vi "RT get system status.vi"(8 "error in (no error)":errorcluster, 9 "FPGA version":string="N/A", 10 "RT Main version":string="N/A", 11 "FPGA VI Reference in":refnum<k20>) -> (0 "error out":errorcluster, 3 "status summary string":string)   [LabVIEW 2018]
uses:
  Message Queue/error queue name (constant).ctl
  <vilib>/Utility/error.llb/Error Cluster From Error Code.vi
  <vilib>/rvi/errors/niLvFpgaAdjustHostInterfaceError.vi
  <vilib>/nisyscfg/Close (System).vi
  Globals/RT AND FPGA SETTINGS.vi
  <vilib>/rvi/interface/nirviReadWriteControl/nirviReadWriteControl.xnode
  <vilib>/NI_Real-Time Target Support.lvlib
  <vilib>/nisyscfg/nisyscfg.lvlib
  Message Queue/Message Queue.lvlib
  <resource>/objmgr/nisysapi.rc
  NiFpgaLv.dll
  <vilib>/rvi/interface/Simulation/niFpgaSimulationCallBeginRW.vi
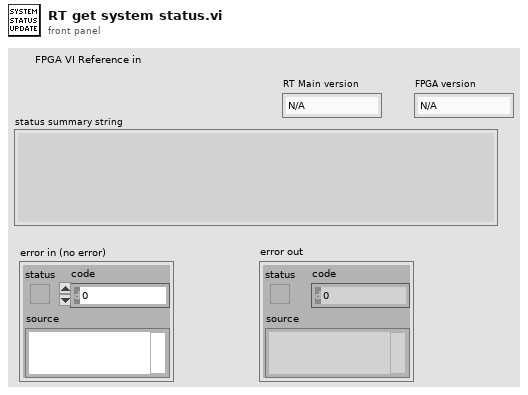
[diagram p1: front panel]
types:
  T1 = typedef "Message Queue.lvlib/error queue name (constant).ctl" = string
  T2 = enum16{"Safe State", "I/O with PID Control", "Fast Output Only", "NOT_READY"}
  T3 = typedef "NI_Real-Time Target Support.lvlib/RT CPU Load.ctl" = cluster{"Total (%)":dbl, "Time Critical (%)":dbl, "Timed Structures (%)":dbl, "High (%)":dbl, "Above Normal (%)":dbl, "Normal (%)":dbl, "Background (%)":dbl, "Idle (%)":dbl, "ISR (%)":dbl}
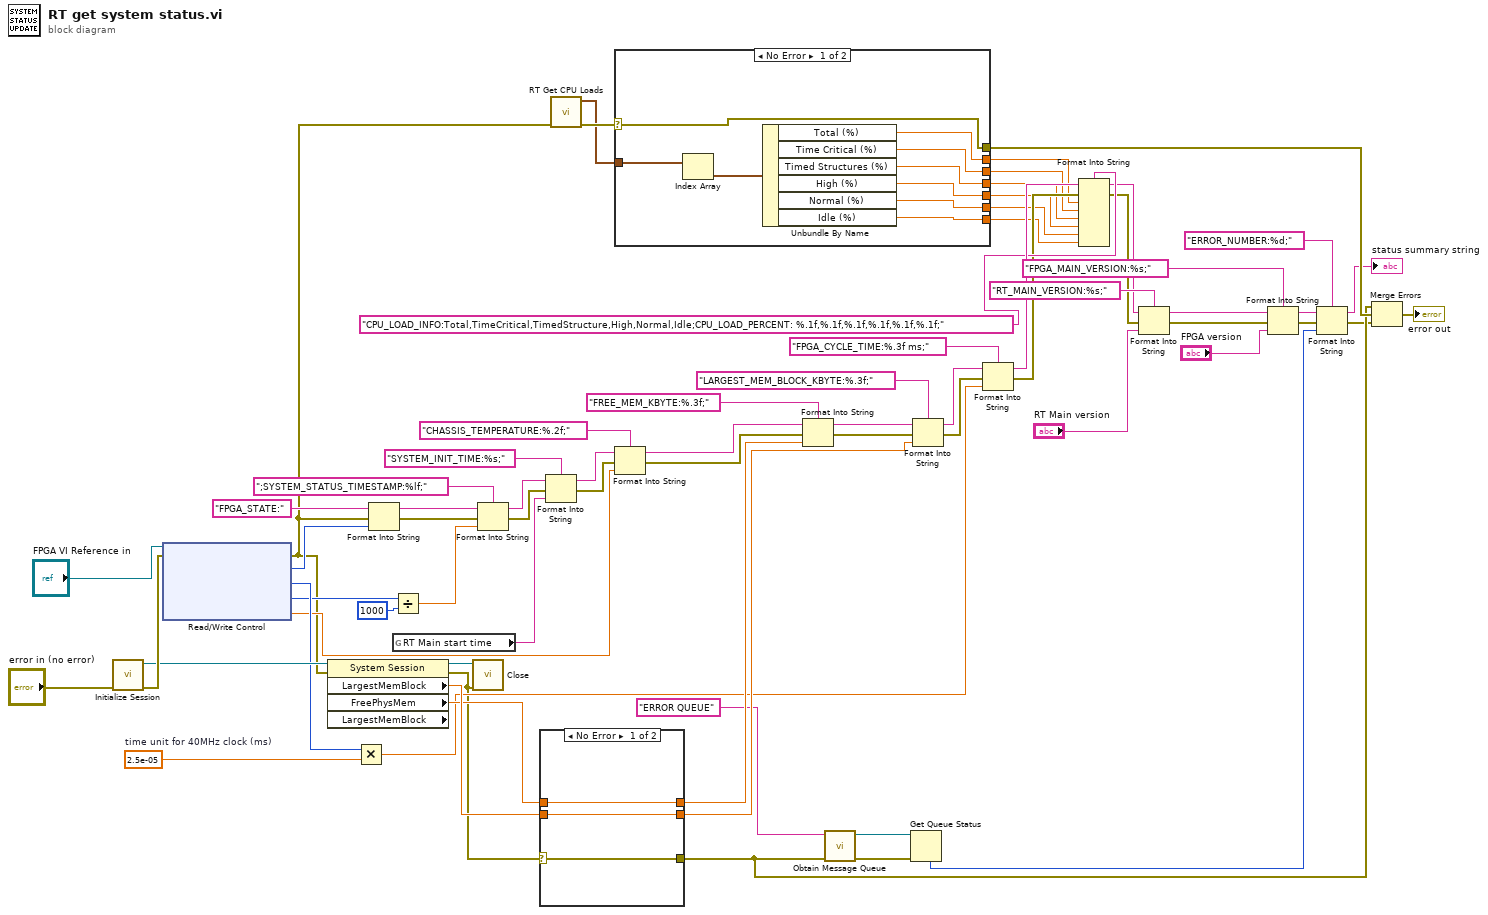
[diagram p0: block diagram]
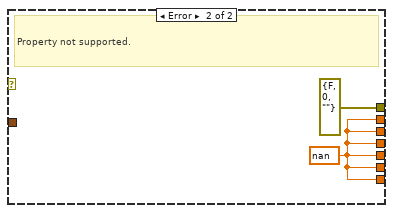
[diagram p2: hidden frame]
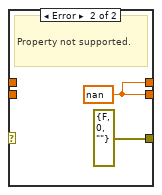
[diagram p3: hidden frame]
diagram:
  w56 = 2.5e-05  # time unit for 40MHz clock (ms)
  n1 = call <vilib>:"Initialize Session.vi"("error in (no error)"="error in (no error)") -> ("error out"=w70:errorcluster, "Session out"=w69:refnum<k21>)  [unwired: 9 in]
  n2 = xnode "Read/Write Control"("FPGA VI Reference In"="FPGA VI Reference in", "error in"=w70) -> ("error out"=w27:errorcluster, "FPGA state"=w65:T2, "ticks"=w57:i64, "time stamp (ms)"=w49:u64, "Chassis Temperature"=w44:sgl)  [unwired: 1 out]
  n3 = property class="System Session" props=["LargestMemBlock", "FreePhysMem", "LargestMemBlock"](reference=w69, error in=w27) -> (reference out=w8:refnum<k21>, error out=w7:errorcluster, "LargestMemBlock"=w67:dbl, "FreePhysMem"=w66:dbl)  [unwired: 1 out]
  n4 = Multiply(x=w57, y=w56) -> (x*y=w55:dbl)
  n5 = Format Into String(initial string="FPGA_STATE:", error in=w27, w65) -> (resulting string=w45:string, error out=w26:errorcluster)  [unwired: 1 in]
  n6 = Divide(x=w49, y=u64 1000) -> (x/y=w47:dbl)
  n7 = global read "RT AND FPGA SETTINGS.vi" "RT Main start time"() -> (w5:string)
  n8 = call-poly <vilib>:"Close.vi"("error in (no error)"=w7, "Session in"=w8) -> ()  [unwired: 9 in, 1 out]
  n9 = Format Into String(format string=";SYSTEM_STATUS_TIMESTAMP:%lf;", initial string=w45, error in=w26, w47) -> (resulting string=w2:string, error out=w4:errorcluster)
  n10 = case shown="No Error" w7 {
    selector: w7 -> [w71 _]
    tunnel: w67 -> [w72 _]
    tunnel: [w72 w75] -> w59
    tunnel: w66 -> [w73 _]
    tunnel: [w73 w75] -> w63
    tunnel: [w71 errorcluster {"status"=FALSE, "code"=0, "source"=""} ("error IO")] -> w33
    frame No Error {
    }
    frame Error {
      w75 = nan
      # "Property not supported."
    }
  }
  n11 = Format Into String(format string="SYSTEM_INIT_TIME:%s;", initial string=w2, error in=w4, w5) -> (resulting string=w1:string, error out=w3:errorcluster)
  n12 = call <vilib>:"RT Get CPU Loads.vi"("error in (no error)"=w27) -> ("error out"=w51:errorcluster, "CPU loads"=w50:T3[])  [unwired: 9 in]
  n13 = case shown="No Error" w51 {
    selector: w51 -> [w84 _]
    tunnel: [w81 w85] -> w15
    tunnel: [w84 errorcluster {"status"=FALSE, "code"=0, "source"=""} ("error IO")] -> w35
    tunnel: w50 -> [w82 _]
    tunnel: [w80 w85] -> w13
    tunnel: [w79 w85] -> w12
    tunnel: [w78 w85] -> w11
    tunnel: [w77 w85] -> w10
    tunnel: [w76 w85] -> w14
    frame No Error {
      n14 = Index Array(array=w82) -> (element=w83:T3)  [unwired: 1 in]
      n15 = Unbundle By Name(w83) -> ("Total (%)"=w81:dbl, "Time Critical (%)"=w76:dbl, "Timed Structures (%)"=w80:dbl, "High (%)"=w79:dbl, "Normal (%)"=w78:dbl, "Idle (%)"=w77:dbl)
    }
    frame Error {
      w85 = nan
      # "Property not supported."
    }
  }
  n16 = Format Into String(format string="CHASSIS_TEMPERATURE:%.2f;", initial string=w1, error in=w3, w44) -> (resulting string=w42:string, error out=w25:errorcluster)
  n17 = Format Into String(format string="FREE_MEM_KBYTE:%.3f;", initial string=w42, error in=w25, w63) -> (resulting string=w61:string, error out=w24:errorcluster)
  n18 = call "Obtain Message Queue.vi"("error in (no error)"=w33, "name (unnamed)"=T1 "ERROR QUEUE" ("Error queue name")) -> ("error out"=w32:errorcluster, "Message Queue"=w31:refnum<queue>)  [unwired: 7 in, 1 out]
  n19 = Get Queue Status(queue=w31, error in (no error)=w32) -> (# elements in queue=w30:i32)  [unwired: 1 in, 7 out]
  n20 = Format Into String(format string="LARGEST_MEM_BLOCK_KBYTE:%.3f;", initial string=w61, error in=w24, w59) -> (resulting string=w58:string, error out=w23:errorcluster)
  n21 = Format Into String(format string="FPGA_CYCLE_TIME:%.3f ms;", initial string=w58, error in=w23, w55) -> (resulting string=w53:string, error out=w22:errorcluster)
  n22 = Format Into String(format string="CPU_LOAD_INFO:Total,TimeCritical,TimedStructure,High,Normal,Idle;CPU_LOAD_PERCENT: %.1f,%.1f,%.1f,%.1f,%.1f,%.1f;", initial string=w53, error in=w22, w15, w14, w13, w12, w11, w10) -> (resulting string=w37:string, error out=w21:errorcluster)
  n23 = Format Into String(format string="RT_MAIN_VERSION:%s;", initial string=w37, error in=w21, "RT Main version") -> (resulting string=w36:string, error out=w20:errorcluster)
  n24 = Format Into String(format string="FPGA_MAIN_VERSION:%s;", initial string=w36, error in=w20, "FPGA version") -> (resulting string=w28:string, error out=w19:errorcluster)
  n25 = Format Into String(format string="ERROR_NUMBER:%d;", initial string=w28, error in=w19, w30) -> (resulting string=→"status summary string":string, error out=w18:errorcluster)
  n26 = Merge Errors(w33, w35, w18) -> (→"error out":errorcluster)
